vi "ReadingsIntoCSVData.vi"(0 "Fridge Temoerature":dbl format="%#.1g", 1 "Wine Cellar Temperature":dbl, 2 "Greenhouse Temperature":dbl, 3 "Greenhouse VPD":dbl, 4 "Greenhouse PAR":u16) -> (5 "Array":string[](array[string]))   [LabVIEW 2019]
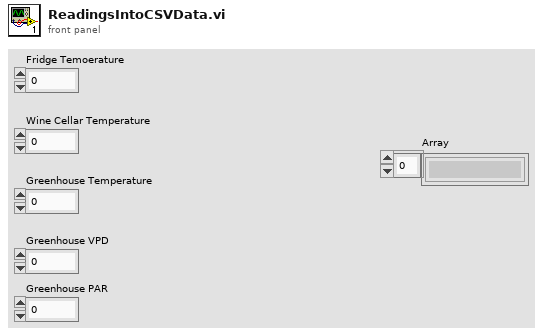
[diagram p1: front panel]
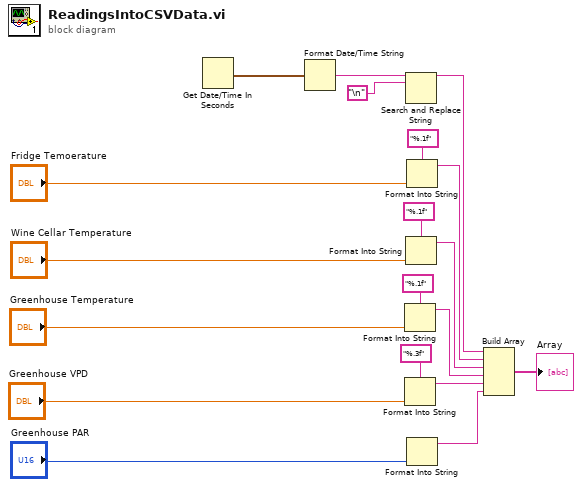
[diagram p0: block diagram]
diagram:
  n1 = Get Date/Time In Seconds() -> (seconds since 1Jan1904=w19:timestamp)
  n2 = Format Date/Time String(seconds (now)=w19) -> (date/time string=w18:string)  [unwired: 2 in]
  n3 = Format Into String(format string="%.1f", "Greenhouse Temperature") -> (resulting string=w9:string)  [unwired: 2 in, 1 out]
  n4 = Format Into String(format string="%.3f", "Greenhouse VPD") -> (resulting string=w8:string)  [unwired: 2 in, 1 out]
  n5 = Search and Replace String(input string=w18, search string="\n") -> (result string=w17:string)  [unwired: 6 in, 3 out]
  n6 = Format Into String(format string="%.1f", "Wine Cellar Temperature") -> (resulting string=w12:string)  [unwired: 2 in, 1 out]
  n7 = Format Into String(format string="%.1f", "Fridge Temoerature") -> (resulting string=w13:string)  [unwired: 2 in, 1 out]
  n8 = Format Into String("Greenhouse PAR") -> (resulting string=w6:string)  [unwired: 3 in, 1 out]
  n9 = Build Array(w17, w13, w12, w9, w8, w6) -> (→"Array":string[])
